vi "FGV servo initialized.vi"(8 "Write?(F)":bool, 11 "Initialized in":bool) -> (3 "Initialized out":bool)   [LabVIEW 2017, in "Servo drive module.lvlib"]
doc: "Functonal global variable, whitch holds information, if magnet module is initialized.\nInputs: Initialized in - use true if magnet module was initialized, use false in the begin/end of application.\nWrite - needs to be true for writing into variable, default value is false which will cause only \"read\" functionality\nOutput: Initialized out - Indicates that module was initialized and is ready to follow orders"
uses:
  Servo drive module.lvlib
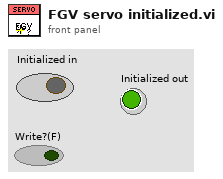
[diagram p1: front panel]
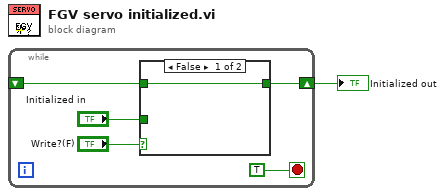
[diagram p0: block diagram]
diagram:
  n1 = while {
    shift-right: [w5] -> w1
    shift-left: _ -> [w4]
    stop <- TRUE stop-if-true
    n2 = case shown="False" "Write?(F)" {
      tunnel: "Initialized in" -> [_ w8]
      tunnel: [w7 w8] -> w5
      tunnel: w4 -> [w7 _]
      frame False {
      }
      frame True {
      }
    }
  }
  "Initialized out" <- w1
